vi "TESTE.vi"() -> ()   [LabVIEW 2018]
panel:
  out "number 2":i32
  out "number":i32
  out "error out":errorcluster
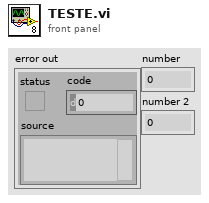
[diagram p1: front panel]
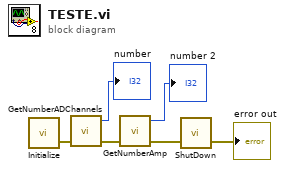
[diagram p0: block diagram]
diagram:
  n1 = call <userlib>:"Initialize.vi"() -> ("error out"=w5:errorcluster)  [unwired: 2 in, 1 out]
  n2 = call <userlib>:"GetNumberADChannels.vi"("error in (no error)"=w5) -> ("error out"=w4:errorcluster, "number"=→"number":i32)  [unwired: 2 in, 1 out]
  n3 = call <userlib>:"GetNumberAmp.vi"("error in (no error)"=w4) -> ("error out"=w3:errorcluster, "number"=→"number 2":i32)  [unwired: 2 in, 1 out]
  n4 = call <userlib>:"ShutDown.vi"("error in (no error)"=w3) -> ("error out"=→"error out":errorcluster)  [unwired: 1 in, 1 out]
